vi "Std_Bus_Initialize.vi"(0 "Communications Port":refnum<visa-resource-name>="COM3", 2 "InterfaceType":i32(ring)=1 items=["Usb", "Serial", "Ethernet", "Unconnected"], 5 "error in (no error)":errorcluster) -> (12 "IsConnected":bool, 14 "ILabVIEW":refnum<k24>, 19 "error out":errorcluster)   [LabVIEW 2018]
doc: "Establishes communication with the <B>Watlow Standard Bus</B> product. Call this VI before calling other instrument driver VIs for this product. Generally, you need to call the <B>Initialize VI</B> only once at the beginning of an application.\n\nThis VI Driver set supports the following communication protocols. The user will select the type from the <B> InterfaceType</B> Control.\n\n<B>Serial</B> - RS 485 Communications - The user will select the serial comms port available in the Communicaitons Port Control (COM3, COM4)\n<B> USB </B> - The user will enter the Unit Serial Number in the Communications Control (Example: 12345). Currently no Watlow products support this protocol. Contact Watlow for avabilabity.\n<B> Ethernet</B> - The user will enter the controls IP address in the Communications Port Control. (Example: 192.168.0.222).\n\n<B> IsConnected</B> control tells the user that a successful communication connection has been established and may continue with any read/write operations. Use this control as an indication that the VI properly initialized.\n<B> Interface Found </B> control tells the user that the selected Interface was found. This does not indicate that it connected to the device. Use the <B> IsConnected </B> control as an indication that the VI properly initialized."
uses:
  C:/RageATE/Instruments/Ess Temp Plate/LabView Driver/Public/Watbus.dll
  Watbus.dll
  <vilib>/regexp/Match Regular Expression.xnode
panel:
  out "Description":string
  out "size(s)":i32
  out "Interface":i32
  # "Std Bus Initialize"
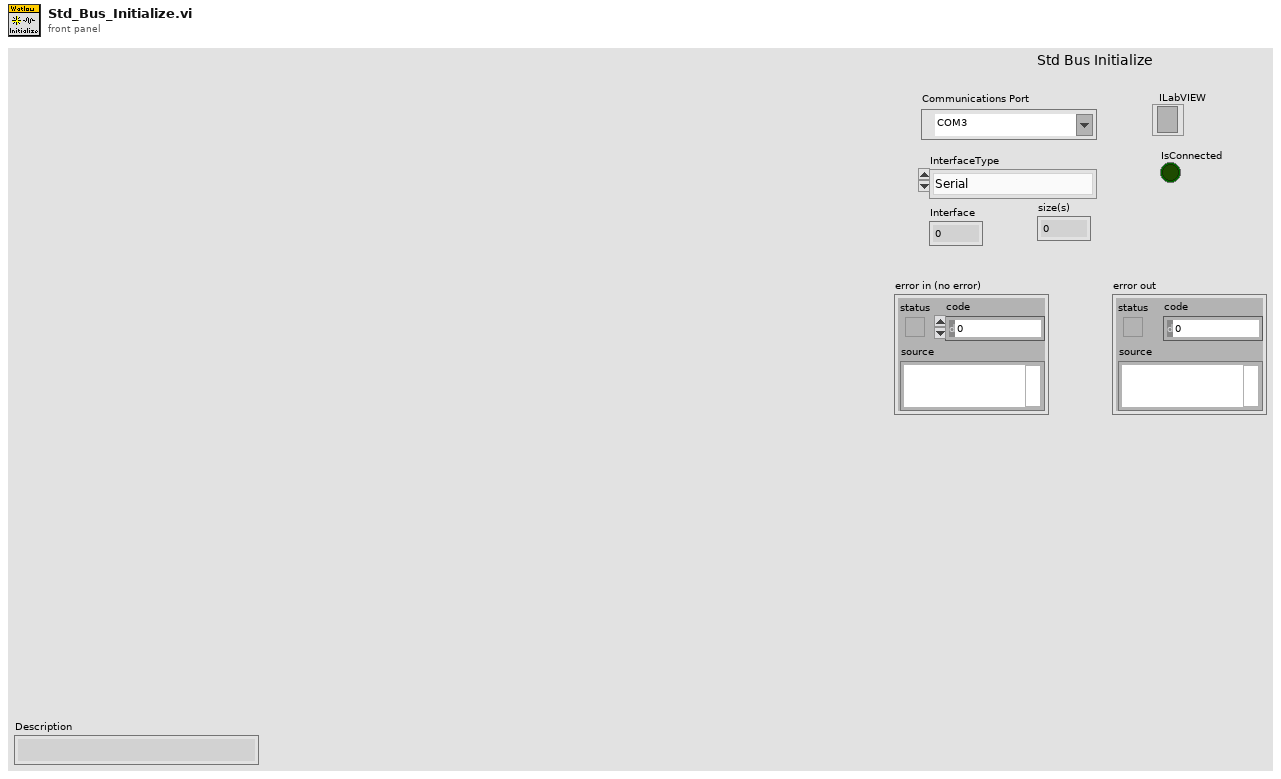
[diagram p1: front panel]
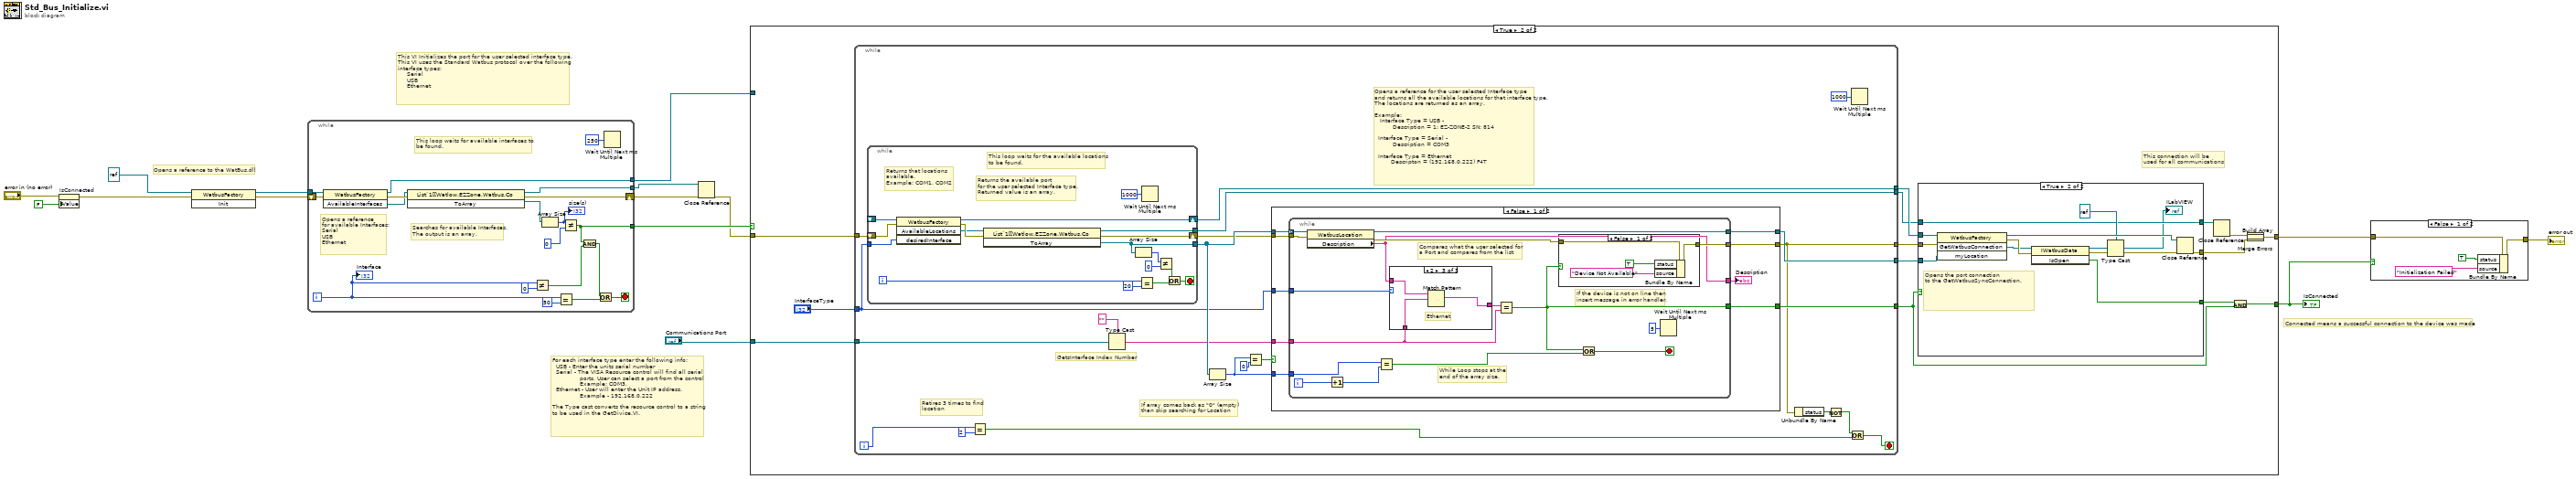
[diagram p0: block diagram]
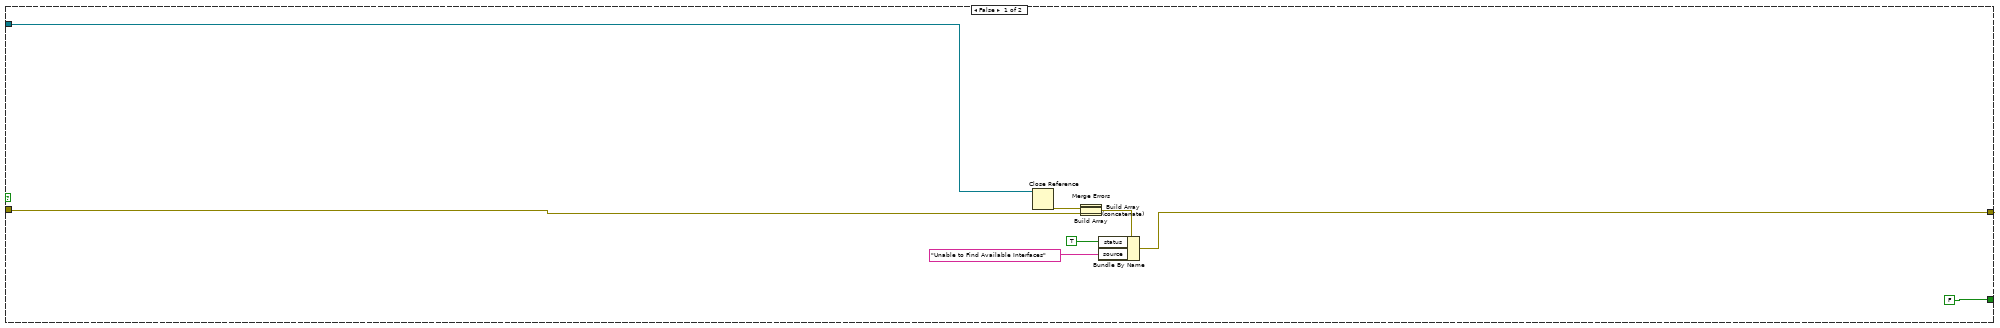
[diagram p3: hidden frame]
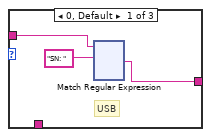
[diagram p4: hidden frame]
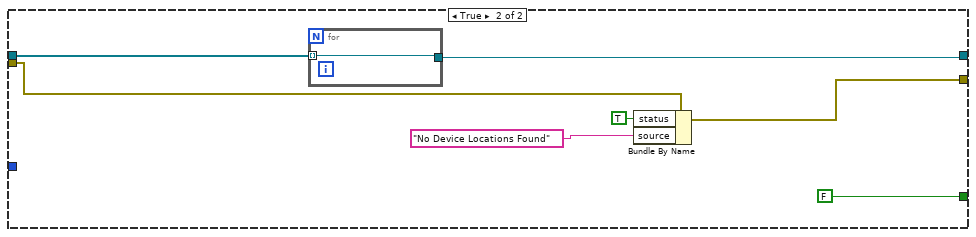
[diagram p7: hidden frame]
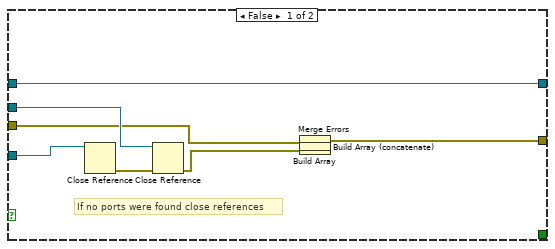
[diagram p8: hidden frame]
diagram:
  # "Opens a reference to the WatBus.dll"
  # "For each interface type enter the following info;\n  USB - Enter the units serial number\n  Serial - The VISA Resource control will find all serial\n               ports. User can select a port from the control\n               Example: COM3.\n  Ethernet - User will enter the Unit IP address.\n               Example - 192.168.0.222\n\nThe Type cast converts the resource control to a string\nto be used in the GetDivice.VI."
  # "Connected means a successful connection to the device was made"
  # "This VI Initializes the port for the user selected interface type.\nThis VI uses the Standard Watbus protocol over the following\ninterface types;\n     Serial\n     USB\n     Ethernet"
  n1 = property on="IsConnected" class="Bool (strict)"(error in="error in (no error)", "Value"=FALSE ("IsConnected")) -> (error out=w14:errorcluster)  [unwired: 1 in, 1 out]
  n2 = invoke class="WatbusFactory" method="Init"(reference=refnum<k24> refnum ("ConstructClient"), error in=w14) -> (reference out=w10:refnum<k24>, error out=w9:errorcluster)  [unwired: 1 in, 1 out]
  n3 = while {
    shift-right: [w28] -> w12
    shift-left: w9 -> [w32]
    tunnel: [w18] -> w8
    tunnel: w10 -> [w33]
    tunnel: [w34] -> w6
    tunnel: [w16] -> w11
    i -> [w24]
    stop <- w21 stop-if-true
    # "This loop waits for available interfaces to \nbe found."
    # "Opens a reference\nfor available Interfaces:\nSerial\nUSB\nEthernet"
    # "Searches for available Interfaces.\nThe output is an array."
    n4 = invoke class="WatbusFactory" method="AvailableInterfaces"(reference=w33, error in=w32) -> (reference out=w34:refnum<k24>, error out=w30:errorcluster, "AvailableInterfaces"=w29:refnum<k24>)  [unwired: 1 in]
    n5 = invoke class="List`1[[Watlow.EZZone.Watbus.Co" method="ToArray"(reference=w29, error in=w30) -> (reference out=w16:refnum<k24>, error out=w28:errorcluster, "ToArray"=w17:refnum<k24>[])  [unwired: 1 in]
    n6 = Not Equal?(x=w24, y=0) -> (x != y?=w25:bool)
    n7 = Array Size(array=w17) -> (size(s)=w19:i32)
    "size(s)" <- w19
    n8 = Equal?(x=w24, y=50) -> (x = y?=w23:bool)
    n9 = Not Equal?(x=w19, y=0) -> (x != y?=w18:bool)
    n10 = And(x=w18, y=w25) -> (x .and. y?=w27:bool)
    n11 = Or(x=w27, y=w23) -> (x .or. y?=w21:bool)
    n12 = Wait Until Next ms Multiple(millisecond multiple=u32 250) -> ()  [unwired: 1 out]
    "Interface" <- w24
  }
  n13 = Close Reference(reference=w11, error in (no error)=w12) -> (error out=w7:errorcluster)
  n14 = case shown="True" w8 {
    tunnel: [w37 w52] -> w2
    tunnel: w7 -> [w38 w51]
    tunnel: w6 -> [w39 _]
    tunnel: [FALSE ("IsOpen") w45] -> w3
    tunnel: "Communications Port" -> [_ w50]
    frame False {
      n15 = Close Reference(reference=w39) -> (error out=w40:errorcluster)  [unwired: 1 in]
      n16 = Build Array(w40, w38) -> (w44:errorcluster[])
      n17 = Build Array (concatenate)(w44) -> (w35:errorcluster[])
      n18 = Merge Errors(w35) -> (w41:errorcluster)
      n19 = Bundle By Name(cluster=w41, "status"=TRUE, "source"="Unable to Find Available Interfaces") -> (w37:errorcluster)
    }
    frame True {
      # "This connection will be\nused for all communications"
      n20 = while {
        tunnel: [w81] -> w59
        tunnel: [w67] -> w58
        tunnel: [w80] -> w57
        tunnel: [w74] -> w54
        tunnel: w51 -> [w73]
        tunnel: w50 -> [w70]
        tunnel: "InterfaceType" -> [w69]
        tunnel: [w68] -> w46
        i -> [w60]
        stop <- w63 stop-if-true
        # "Retires 3 times to find\nlocation"
        # "GetsInterface Index Number"
        # "If array comes back as \"0\" (empty)\nthan skip searching for Location"
        # "Opens a reference for the user selected Interface type\nand returns all the available locations for that interface type. The locations are returned as an array.\n\nExample:\n   Interface Type = USB -\n          Description = 1: EZ-ZONE-2 SN: 814\n\n  Interface Type = Serial -\n          Description = COM3\n\n  Interface Type = Ethernet\n         Descripton = (192.168.0.222) F4T"
        n21 = while {
          tunnel: w69 -> [w242]
          tunnel: [w252] -> w79
          shift-right: [w253] -> w81
          shift-left: _ -> [w255]
          shift-right: [w254] -> w75
          shift-left: w73 -> [w249]
          tunnel: [w241] -> w74
          i -> [w245]
          stop <- w247 stop-if-true
          # "This loop waits for the available locations \nto be found."
          # "Returns that locations\navailable.\nExample; COM1, COM2"
          # "Returns the available port\nfor the user selected Interface type.\nReturned value is an array."
          n22 = invoke class="WatbusFactory" method="AvailableLocations"(reference=w255, error in=w249, "desiredInterface"=w242) -> (reference out=w253:refnum<k24>, error out=w257:errorcluster, "AvailableLocations"=w256:refnum<k24>)  [unwired: 1 in, 1 out]
          n23 = invoke class="List`1[[Watlow.EZZone.Watbus.Co" method="ToArray"(reference=w256, error in=w257) -> (reference out=w241:refnum<k24>, error out=w254:errorcluster, "ToArray"=w252:refnum<k24>[])  [unwired: 1 in]
          n24 = Array Size(array=w252) -> (size(s)=w250:i32)
          n25 = Equal?(x=w245, y=20) -> (x = y?=w244:bool)
          n26 = Wait Until Next ms Multiple(millisecond multiple=u32 1000) -> ()  [unwired: 1 out]
          n27 = Not Equal?(x=w250, y=0) -> (x != y?=w248:bool)
          n28 = Or(x=w248, y=w244) -> (x .or. y?=w247:bool)
        }
        n29 = Equal?(x=w60, y=2) -> (x = y?=w62:bool)
        n30 = Type Cast(type="", x=w70) -> (*(type *) &x=w71:string)
        n31 = Array Size(array=w79) -> (size(s)=w78:i32)
        n32 = Equal?(x=w78, y=0) -> (x = y?=w76:bool)
        n33 = case shown="False" w76 {
          tunnel: [w84 w239] -> w67
          tunnel: [w90 w233] -> w80
          tunnel: w75 -> [w89 w238]
          tunnel: w69 -> [w88 _]
          tunnel: w78 -> [w87 _]
          tunnel: w79 -> [w86 w234]
          tunnel: [w85 FALSE] -> w68
          tunnel: w71 -> [w82 _]
          frame False {
            n34 = while {
              tunnel: w89 -> [w106]
              tunnel: w86 -> [w105] mode=indexing
              tunnel: w87 -> [w100]
              tunnel: w88 -> [w99]
              tunnel: [w97] -> w90
              tunnel: [w95] -> w85
              tunnel: [w93] -> w84
              tunnel: [w92] -> w83
              tunnel: w82 -> [w91]
              i -> [w101]
              stop <- w94 stop-if-true
              # "Compares what the user selected for\na Port and compares from the list"
              # "If the device is not on line then\ninsert message in error handler."
              # "While Loop stops at the\nend of the array size."
              n35 = property class="WatbusLocation"(reference=w105, error in=w106) -> (reference out=w97:refnum<k24>, error out=w102:errorcluster, "Description"=w92:string)
              n36 = Increment(x=w101) -> (x+1=w103:i32)
              n37 = Equal?(x=w100, y=w103) -> (x = y?=w104:bool)
              n38 = case shown="2" w99 {
                tunnel: w92 -> [w108 w224 w227]
                tunnel: [w107 w224 w225] -> w98
                tunnel: w91 -> [_ _ w226]
                frame 0, Default {
                  # "USB"
                  n39 = xnode "Match Regular Expression"("input string"=w108, "regular expression"="SN: ") -> ("after match"=w107:string)  [unwired: 2 in, 6 out]
                }
                frame 1 {
                  # "Serial Comms"
                }
                frame 2 {
                  # "Ethernet"
                  n40 = Match Pattern(string=w227, regular expression=w226) -> (match substring=w225:string)  [unwired: 4 out]
                }
              }
              n41 = Equal?(x=w98, y=w91) -> (x = y?=w95:bool)
              n42 = case shown="False" w95 {
                tunnel: w102 -> [w231 w232]
                tunnel: [w230 w232] -> w93
                frame False {
                  n43 = Bundle By Name(cluster=w231, "status"=TRUE, "source"="Device Not Available") -> (w230:errorcluster)
                }
                frame True {
                }
              }
              n44 = Or(x=w95, y=w104) -> (x .or. y?=w94:bool)
              n45 = Wait Until Next ms Multiple(millisecond multiple=u32 5) -> ()  [unwired: 1 out]
            }
            "Description" <- w83
          }
          frame True {
            n46 = for {
              tunnel: w234 -> [w240] mode=indexing
              tunnel: [w240] -> w233
            }
            n47 = Bundle By Name(cluster=w238, "status"=TRUE, "source"="No Device Locations Found") -> (w239:errorcluster)
          }
        }
        n48 = Unbundle By Name(w67) -> ("status"=w65:bool)
        n49 = Not(x=w65) -> (.not. x?=w64:bool)
        n50 = Or(x=w64, y=w62) -> (x .or. y?=w63:bool)
        n51 = Wait Until Next ms Multiple(millisecond multiple=u32 1000) -> ()  [unwired: 1 out]
      }
      n52 = case shown="True" w46 {
        tunnel: [w263 w278] -> w55
        tunnel: w59 -> [w266 w277]
        tunnel: w58 -> [w265 w276]
        tunnel: w57 -> [w262 w275]
        tunnel: w54 -> [w259 w270]
        tunnel: [w259 w270] -> w53
        tunnel: [_ w268] -> w47
        frame False {
          # "If no ports were found close references"
          n53 = Close Reference(reference=w262) -> (error out=w261:errorcluster)  [unwired: 1 in]
          n54 = Close Reference(reference=w266, error in (no error)=w261) -> (error out=w264:errorcluster)
          n55 = Build Array(w265, w264) -> (w260:errorcluster[])
          n56 = Build Array (concatenate)(w260) -> (w258:errorcluster[])
          n57 = Merge Errors(w258) -> (w263:errorcluster)
        }
        frame True {
          # "Opens the port connection\nto the GetWatbusSyncConnection."
          n58 = invoke class="WatbusFactory" method="GetWatbusConnection"(reference=w277, error in=w276, "myLocation"=w275) -> (reference out=w279:refnum<k24>, error out=w274:errorcluster, "GetWatbusConnection"=w273:refnum<k24>)  [unwired: 1 in, 1 out]
          n59 = invoke class="IWatbusData" method="IsOpen"(reference=w273, error in=w274) -> (reference out=w272:refnum<k24>, error out=w269:errorcluster, "IsOpen"=w268:bool)  [unwired: 1 in]
          n60 = Type Cast(type=refnum<k24> refnum ("ConstructClient"), x=w272) -> (*(type *) &x=→"ILabVIEW":refnum<k24>)
          n61 = Close Reference(reference=w279, error in (no error)=w269) -> (error out=w278:errorcluster)
        }
      }
      n62 = Close Reference(reference=w53) -> (error out=w56:errorcluster)  [unwired: 1 in]
      n63 = And(x=w47, y=w46) -> (x .and. y?=w45:bool)
      n64 = Build Array(w56, w55) -> (w48:errorcluster[])
      n65 = Merge Errors(w48) -> (w52:errorcluster)
    }
  }
  "IsConnected" <- w3
  n66 = case shown="False" w3 {
    tunnel: w2 -> [w283 w284]
    tunnel: [w282 w284] -> w1
    frame False {
      n67 = Bundle By Name(cluster=w283, "status"=TRUE, "source"="Initialization Failed") -> (w282:errorcluster)
    }
    frame True {
    }
  }
  "error out" <- w1
